vi "ProcMsg.vi"(0 "reference in":refnum<class "Proccess.lvclass">, 5 "error in (no error)":errorcluster) -> (14 "reference out":refnum<class "Proccess.lvclass">, 19 "error out":errorcluster)   [LabVIEW 2019, in "Proccess.lvclass"]
uses:
  Proccess.lvclass
  Proccess.lvclass/Proccess.ctl
  MessageInterface_class/MessageInterface.lvclass
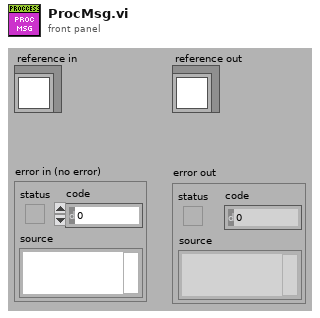
[diagram p1: front panel]
types:
  T1 = typedef "MessageInterface.lvclass/Message.ctl" = cluster{"name":string, "value":string, "receiver host":string, "receiver process":string, "source host":string, "source process":string}
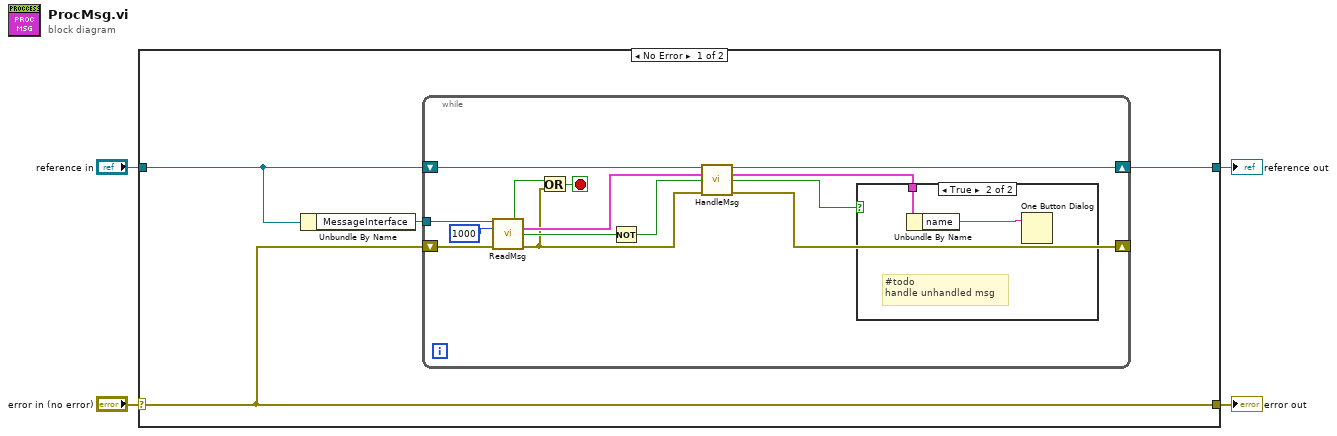
[diagram p0: block diagram]
diagram:
  n1 = case shown="No Error" "error in (no error)" {
    selector: "error in (no error)" -> [w8 w26]
    tunnel: [w8 w26] -> w3
    tunnel: [w5 w25] -> w1
    tunnel: "reference in" -> [w7 w25]
    frame No Error {
      n2 = Unbundle By Name(w7) -> ("MessageInterface"=w6:refnum<class "MessageInterface.lvclass">)
      n3 = while {
        shift-right: [w17] -> w5
        shift-left: w7 -> [w18]
        tunnel: w6 -> [w22]
        shift-right: [w16] -> _
        shift-left: w8 -> [w20]
        stop <- w11 stop-if-true
        n4 = call-dynamic "ReadMsg.vi"("reference in"=w22, "timeout (10 s)"=1000 ("timeout (1 ms)"), "error in (no error)"=w20) -> ("exit process?"=w19:bool, "message"=w15:T1, "timed out?"=w12:bool, "error out"=w10:errorcluster)  [unwired: 8 in, 1 out]
        n5 = Or(x=w19, y=w10) -> (x .or. y?=w11:bool)
        n6 = Not(x=w12) -> (.not. x?=w14:bool)
        n7 = call-dynamic "HandleMsg.vi"("reference in"=w18, "message in"=w15, "Unhandled in"=w14, "error in (no error)"=w10) -> ("reference out"=w17:refnum<class "Proccess.lvclass">, "message out"=w9:T1, "Unhandled out"=w13:bool, "error out"=w16:errorcluster)  [unwired: 8 in]
        n8 = case shown="True" w13 {
          tunnel: w9 -> [_ w24]
          frame False {
          }
          frame True {
            # "#todo\nhandle unhandled msg"
            n9 = Unbundle By Name(w24) -> ("name"=w23:string)
            n10 = One Button Dialog(message=w23) -> ()  [unwired: 1 in, 1 out]
          }
        }
      }
    }
    frame Error {
    }
  }
  "error out" <- w3
  "reference out" <- w1
